vi "Run Scoring Async.vi"(4 "Server":refnum<class "SOL-Server.lvclass">, 5 "Submission DB":refnum<class "Submission DB.lvclass">, 7 "Submission":refnum<class "Submission.lvclass">, 9 "Scorer Path":path, 10 "LLB Path":path, 11 "Scorer in":refnum<class "Scorer.lvclass">) -> ()   [LabVIEW 2020, in "Summer of LabVIEW.lvlib" / "Scorer.lvclass"]
uses:
  Scorer.lvclass
  Submission/Submission.lvclass
  SOL-Server/SOL-Server.lvclass
  Submission DB/Submission DB.lvclass
panel:
  out "return code":i32
  out "standard output":string
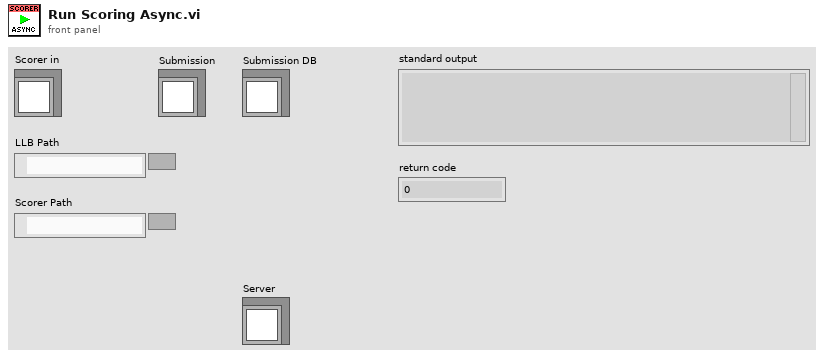
[diagram p1: front panel]
types:
  T1 = typedef "SoL Scoring.lvlib/Score.ctl" = cluster{"Overall":dbl, "Categories":T2[]}
  T2 = typedef "SoL Scoring.lvlib/Score Entry.ctl" = cluster{"Category":string, "Value":dbl}
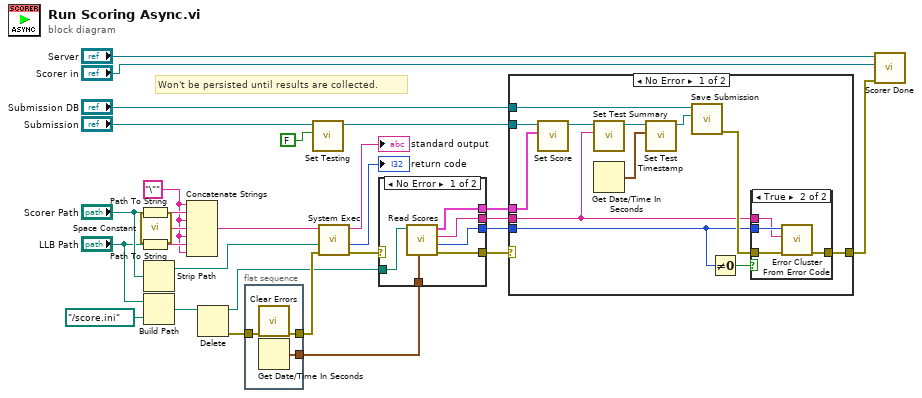
[diagram p0: block diagram]
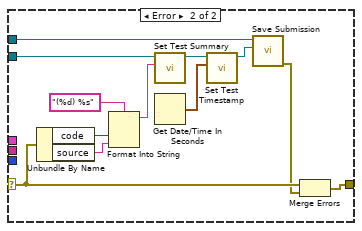
[diagram p3: hidden frame]
diagram:
  w25 = "\""
  # "Won't be persisted until results are collected."
  n1 = Path To String(path="Scorer Path") -> (string=w28:string)
  n2 = Path To String(path="LLB Path") -> (string=w26:string)
  n3 = call <vilib>:"Space Constant.vi"() -> ("String"=w27:string)
  n4 = Strip Path(path="Scorer Path") -> (stripped path=w22:path)  [unwired: 1 out]
  n5 = Build Path(base path="LLB Path", name or relative path=path "../score.ini") -> (appended path=w8:path)
  n6 = Concatenate Strings(w25, w28, w25, w27, w25, w26, w25) -> (w24:string)
  n7 = Delete(path (use dialog)=w8) -> (deleted path=w5:path, error out=w7:errorcluster)  [unwired: 4 in, 1 out]
  n8 = flat-sequence {
    tunnel: w7 -> [w31]
    tunnel: [w30] -> w6
    tunnel: [w29] -> w4
    frame #0 {
      n9 = call <vilib>:"Clear Errors.vi"("error in (no error)"=w31) -> ("error out"=w30:errorcluster)  [unwired: 5 in, 1 out]
      n10 = Get Date/Time In Seconds() -> (seconds since 1Jan1904=w29:timestamp)
    }
  }
  n11 = call "Set Testing.vi"("Testing"=FALSE, "Submission in"="Submission") -> ("Submission out"=w1:refnum<class "Submission.lvclass">)  [unwired: 9 in]
  n12 = call <vilib>:"System Exec.vi"("error in (no error)"=w6, "working directory"=w22, "command line"=w24) -> ("error out"=w19:errorcluster, "return code"=→"return code":i32, "standard output"=→"standard output":string)  [unwired: 5 in, 1 out]
  n13 = case shown="No Error" w19 {
    selector: w19 -> [_ w38]
    tunnel: w5 -> [w37 _]
    tunnel: [w36 w38] -> w16
    tunnel: [w35 _] -> w13
    tunnel: [w34 _] -> w14
    tunnel: [w33 _] -> w15
    tunnel: w4 -> [w32 _]
    frame No Error {
      n14 = call "Read Scores.vi"("Start Time"=w32, "Score INI"=w37) -> ("error out"=w36:errorcluster, "Error Code"=w33:i32, "Test Summary"=w34:string, "Score"=w35:T1)  [unwired: 6 in]
    }
    frame Error {
    }
  }
  n15 = case shown="No Error" w16 {
    selector: w16 -> [_ w62]
    tunnel: w15 -> [w40 _]
    tunnel: w14 -> [w42 _]
    tunnel: w13 -> [w49 _]
    tunnel: "Submission DB" -> [w47 w65]
    tunnel: w1 -> [w50 w67]
    tunnel: [w41 w60] -> w11
    frame No Error {
      n16 = call "Set Score.vi"("Score"=w49, "Submission in"=w50) -> ("Submission out"=w48:refnum<class "Submission.lvclass">)  [unwired: 8 in, 1 out]
      n17 = call "Set Test Summary.vi"("Test Summary"=w42, "Submission in"=w48) -> ("Submission out"=w46:refnum<class "Submission.lvclass">)  [unwired: 8 in, 1 out]
      n18 = Get Date/Time In Seconds() -> (seconds since 1Jan1904=w45:timestamp)
      n19 = call "Set Test Timestamp.vi"("Test Timestamp"=w45, "Submission in"=w46) -> ("Submission out"=w44:refnum<class "Submission.lvclass">)  [unwired: 8 in, 1 out]
      n20 = call "Save Submission.vi"("Submission"=w44, "Submission DB in"=w47) -> ("error out"=w43:errorcluster)  [unwired: 8 in, 1 out]
      n21 = Not Equal To 0?(x=w40) -> (x != 0?=w39:bool)
      n22 = case shown="True" w39 {
        tunnel: w43 -> [w51 w55]
        tunnel: w40 -> [_ w54]
        tunnel: w42 -> [_ w53]
        tunnel: [w51 w52] -> w41
        frame False {
        }
        frame True {
          n23 = call <vilib>:"Error Cluster From Error Code.vi"("error in (no error)"=w55, "error message (\"\")"=w53, "error code (0)"=w54) -> ("error out"=w52:errorcluster)  [unwired: 6 in]
        }
      }
    }
    frame Error {
      n24 = Unbundle By Name(w62) -> ("code"=w58:i32, "source"=w57:string)
      n25 = Format Into String(format string="(%d) %s", w58, w57) -> (resulting string=w56:string)  [unwired: 2 in, 1 out]
      n26 = call "Set Test Summary.vi"("Test Summary"=w56, "Submission in"=w67) -> ("Submission out"=w63:refnum<class "Submission.lvclass">)  [unwired: 8 in, 1 out]
      n27 = Get Date/Time In Seconds() -> (seconds since 1Jan1904=w66:timestamp)
      n28 = call "Set Test Timestamp.vi"("Test Timestamp"=w66, "Submission in"=w63) -> ("Submission out"=w64:refnum<class "Submission.lvclass">)  [unwired: 8 in, 1 out]
      n29 = call "Save Submission.vi"("Submission"=w64, "Submission DB in"=w65) -> ("error out"=w61:errorcluster)  [unwired: 8 in, 1 out]
      n30 = Merge Errors(w62, w61) -> (w60:errorcluster)
    }
  }
  n31 = call "Scorer Done.vi"("error in (no error)"=w11, "Scorer"="Scorer in", "SOL-Server in"="Server") -> ()  [unwired: 7 in, 2 out]
